vi "Generate Frame Pulse.vi"(11 "Neopixel - FPGA In":refnum<class "Neopixel - FPGA.lvclass">) -> (1 "Done":bool, 2 "Pulse Output":bool, 3 "Neopixel - FPGA Out":refnum<class "Neopixel - FPGA.lvclass">)   [LabVIEW 2021, in "Neopixel - FPGA.lvclass"]
uses:
  Neopixel - FPGA.lvclass
  Neopixel - FPGA.lvclass/Neopixel - FPGA.ctl
  <vilib>/rvi/DataTransferAndStorage/Container/Common/niFpgaContainerExecOnDevCompGetState.vi
  <vilib>/rvi/Emulation/niFpgaEmulationIsFPGAContextNoSignature.vi
  <vilib>/rvi/DataTransferAndStorage/Container/Common/niFpgaContainerGetUniqueNameForEmu.vi
  <vilib>/rvi/Emulation/niFpgaProcessEmulError.vi
  <vilib>/rvi/Emulation/niFpgaSctlEmulationGetInTimedLoop.vi
  <vilib>/rvi/errors/nirviReportUnexpectedCaseInternalError (U32).vi
  <vilib>/rvi/Memory/Memory_Emulation/niFpgaMemoryEmulationCacheClearOnFirstRun.vi
  <vilib>/rvi/Memory/Memory_Emulation/nirvimemoryEmulationManagerCache_MakeExclusive.vi
  <vilib>/rvi/Memory/Memory_Emulation/niFpgaMemoryEmulationValidateCache.vi
  <vilib>/rvi/Memory/Memory_Emulation/nirvimemoryEmulationManagerCache_InsertValue.vi
  <vilib>/Utility/error.llb/Clear Errors.vi
  <vilib>/rvi/Memory/Memory_Emulation/nirvimemoryEmulationManagerCache_ReleaseExclusive.vi
  <vilib>/rvi/Memory/Memory_Emulation/nirvimemoryEmulationManagerCache_GetValue.vi
  <vilib>/rvi/Memory/Memory_Emulation/nirvimemoryEmulationManagerCache_SetValue.vi
  <vilib>/rvi/Emulation/niFpgaSctlEmulationResourceMgr.vi
  <vilib>/rvi/DataTransferAndStorage/Container/XNode/niFpgaContainer.xnode
  Controls/Raw Frame Memory.ctl
  <vilib>/rvi/Memory/Memory_Emulation/niFpgaMemoryEmulationRefIn.vi
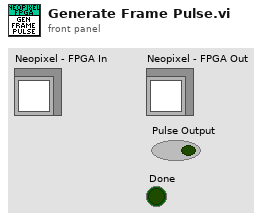
[diagram p1: front panel]
types:
  T1 = typedef "Neopixel - FPGA.lvclass/Raw Frame Memory.ctl" = refnum<k21>
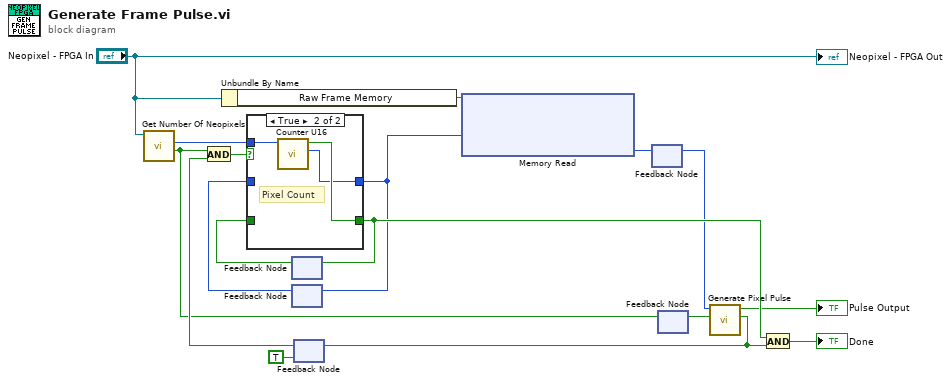
[diagram p0: block diagram]
diagram:
  n1 = call "Get Number Of Neopixels.vi"("Neopixel - FPGA In"="Neopixel - FPGA In") -> ("Valid"=w2:bool, "Number Of Neopixels"=w5:u16)  [unwired: 8 in, 1 out]
  n2 = Unbundle By Name("Neopixel - FPGA In") -> ("Raw Frame Memory"=w11:T1)
  n3 = feedback #1() -> (w15:bool)  [unwired: 1 in]
  n4 = feedback #2() -> (w9:u16)  [unwired: 1 in]
  n5 = feedback #3(TRUE) -> (w4:bool)
  n6 = And(x=w2, y=w4) -> (x .and. y?=w3:bool)
  n7 = case shown="True" w3 {
    tunnel: [w19 w22] -> w16
    tunnel: w15 -> [w19 _]
    tunnel: w5 -> [_ w21]
    tunnel: [w18 w20] -> w10
    tunnel: w9 -> [w18 _]
    frame False {
    }
    frame True {
      # "Pixel Count"
      n8 = call "Counter U16.vi"("Count To"=w21) -> ("Current Value"=w20:u16, "Value Reached"=w22:bool)  [unwired: 9 in]
    }
  }
  n9 = feedback-in #1(w16) -> ()
  n10 = feedback-in #2(w10) -> ()
  n11 = xnode ("Memory Read")("Address"=w10, "Memory In"=w11) -> ("Data"=w8:u32)  [unwired: 1 out]
  n12 = feedback #4() -> (w7:u32)  [unwired: 1 in]
  n13 = feedback-in #4(w8) -> ()
  n14 = feedback #5() -> (w1:bool)  [unwired: 1 in]
  n15 = feedback-in #5(w2) -> ()
  n16 = call "Generate Pixel Pulse.vi"("Ready For Output"=w1, "Data"=w7) -> ("Done"=w17:bool, "Pulse Output"=→"Pulse Output":bool)  [unwired: 8 in]
  n17 = feedback-in #3(w17) -> ()
  n18 = And(x=w16, y=w17) -> (x .and. y?=→"Done":bool)
  "Neopixel - FPGA Out" <- "Neopixel - FPGA In"
